vi "Style_IsParagraphStyle.vi"(4 "Style":refnum<k24>) -> (1 "IsParagraphStyle?":bool)   [LabVIEW 2009]
uses:
  C:/Users/François/Documents/Programmation/_ooReport/DLLs/AODL.dll
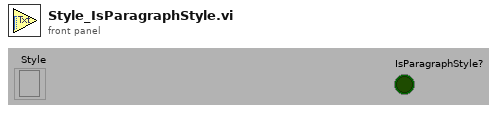
[diagram p1: front panel]
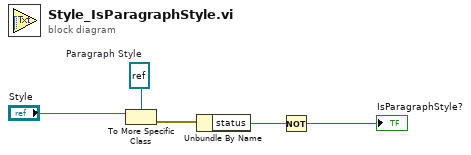
[diagram p0: block diagram]
diagram:
  w5 = refnum<k24> refnum  # Paragraph Style
  n1 = To More Specific Class(target class=w5, reference="Style") -> (error out=w3:errorcluster)  [unwired: 1 in, 1 out]
  n2 = Unbundle By Name(w3) -> ("status"=w2:bool)
  n3 = Not(x=w2) -> (.not. x?=→"IsParagraphStyle?":bool)
